vi "Read.vi"(2 "error in (no error)":errorcluster, 3 "VISA resource name":refnum<visa-resource-name>) -> (0 "read buffer":string, 1 "error out":errorcluster)   [LabVIEW 2011]
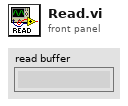
[diagram p1: front panel]
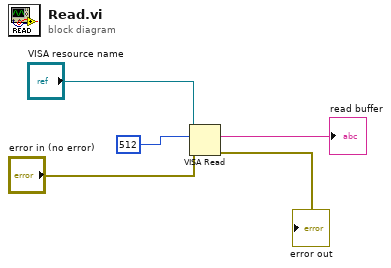
[diagram p0: block diagram]
diagram:
  n1 = VISA Read(VISA resource name="VISA resource name", byte count=u32 512, error in (no error)="error in (no error)") -> (read buffer=→"read buffer":string, error out=→"error out":errorcluster)  [unwired: 2 out]
